vi "Dual Arcade (SubVI).vi"(11 "Joystick Values":dbl[](array[numeric])) -> (2 "Left":dbl, 3 "Right":dbl)   [LabVIEW 2017]
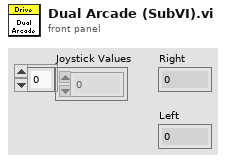
[diagram p1: front panel]
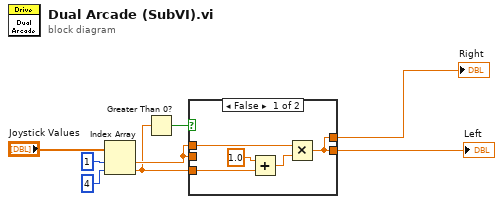
[diagram p0: block diagram]
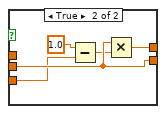
[diagram p2: hidden frame]
diagram:
  n1 = Index Array(array="Joystick Values", index #1=1 ("index"), index #2=4 ("index")) -> (element #1=w8:dbl, element #2=w7:dbl)
  n2 = Greater Than 0?(x=w7) -> (x > 0?=w4:bool)
  n3 = case shown="False" w4 {
    tunnel: w8 -> [_ w17]
    tunnel: [w9 w18] -> w5
    tunnel: [w9 w17] -> w6
    tunnel: w7 -> [w13 w15]
    tunnel: w8 -> [w10 _]
    frame False {
      n4 = Add(x=1.0, y=w13) -> (x+y=w11:dbl)
      n5 = Multiply(x=w10, y=w11) -> (x*y=w9:dbl)
    }
    frame True {
      n6 = Subtract(x=1.0 ("upper limit"), y=w15) -> (x-y=w14:dbl)
      n7 = Multiply(x=w17, y=w14) -> (x*y=w18:dbl)
    }
  }
  "Left" <- w6
  "Right" <- w5
